vi "Find output RPM subvi.vi"(10 "Gear Ratio":dbl, 11 "Motor RPM":dbl) -> (3 "Wheel RPM":dbl)   [LabVIEW 2019]
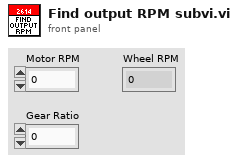
[diagram p1: front panel]
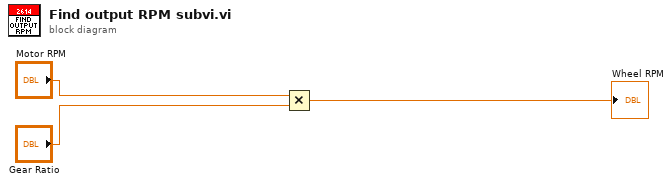
[diagram p0: block diagram]
diagram:
  n1 = Multiply(x="Motor RPM", y="Gear Ratio") -> (x*y=→"Wheel RPM":dbl)
